vi "Untitled 3 (SubVI).vi"(8 "error in (no error)":errorcluster, 10 "Boolean":bool, 11 "VI in":refnum<vi>) -> (0 "error out":errorcluster, 3 "VI out":refnum<vi>)   [LabVIEW 2015]
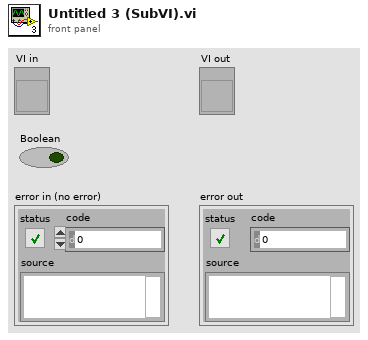
[diagram p1: front panel]
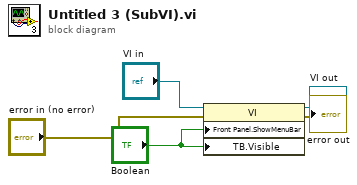
[diagram p0: block diagram]
diagram:
  n1 = property class="VI"(reference="VI in", error in="error in (no error)", "Front Panel.ShowMenuBar"="Boolean", "TB.Visible"="Boolean") -> (reference out=→"VI out":refnum<vi>, error out=→"error out":errorcluster)
